vi "Release UIM.vi"(8 "Error In":errorcluster, 11 "UIM Handle":refnum<data-value>) -> (0 "Error Out":errorcluster)   [LabVIEW 2015, in "UIM.lvclass"]
doc: "Release the obtained reference to the UIM."
uses:
  UIM.lvclass
  UIM.lvclass/UIM.ctl
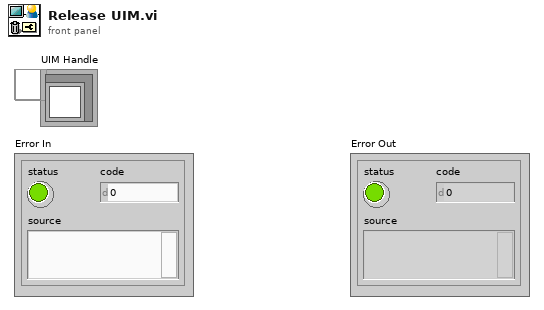
[diagram p1: front panel]
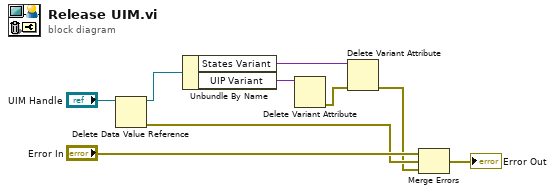
[diagram p0: block diagram]
diagram:
  n1 = Delete Data Value Reference(data value reference="UIM Handle") -> (data value=w7:refnum<class "UIM.lvclass">, error out=w6:errorcluster)  [unwired: 1 in]
  n2 = Unbundle By Name(w7) -> ("States Variant"=w3:variant, "UIP Variant"=w4:variant)
  n3 = Delete Variant Attribute(7:w4) -> (0:w2:errorcluster)  [unwired: 2 in, 2 out]
  n4 = Delete Variant Attribute(4:w2, 7:w3) -> (0:w1:errorcluster)  [unwired: 1 in, 2 out]
  n5 = Merge Errors("Error In", w6, w1) -> (→"Error Out":errorcluster)
